vi "Elevator Controller.vi"(8 "error in":errorcluster) -> ()   [LabVIEW 2017]
doc: "This VI executes continuously carrying out the current operation and responding to updates or new operations. It will often contain the timing or control code that is difficult to place directly in TeleOp. This VI generally opens all sensors and motors and isolates the rest of the robot code from knowing how the operations are carried out."
uses:
  <vilib>/Rock Robotics/WPI/Framework/Completion Status.ctl
  Elevator Setpoints.ctl
  Elevator Operations.ctl
  <vilib>/Rock Robotics/WPI/ThirdParty/Phoenix-LabVIEW/Motor Controller/Controls/CTRE_Phoenix_MotorControl_FeedbackDevice.ctl
  <vilib>/Rock Robotics/WPI/ThirdParty/Phoenix-LabVIEW/Motor Controller/Controls/CTRE_Phoenix_MotorControl_LimitSwitchNormal.ctl
  <vilib>/Rock Robotics/WPI/ThirdParty/Phoenix-LabVIEW/Motor Controller/Controls/CTRE_Phoenix_MotorControl_LimitSwitchSource_Local.ctl
  <vilib>/Rock Robotics/WPI/ThirdParty/Phoenix-LabVIEW/Motor Controller/Controls/CTRE_Phoenix_MotorControl_ControlMode.ctl
  <vilib>/Rock Robotics/WPI/ThirdParty/Phoenix-LabVIEW/Motor Controller/Get/CTRE_Phoenix_MotorController_GetSelectedSensorData.vi
  <vilib>/Rock Robotics/Network Tables/NT Write Boolean.vi
panel:
  out "Position (Raw Sensor Units)":i32
  in  "Acceleration":i32
  in  "Cruise Velocity":i32
  in  "F":dbl
  in  "P":dbl
  in  "I":dbl
  in  "D":dbl
  in  "Interactive Values":T1
  out "Current\nCmd":string
  in  "Buttons":cluster{"Execute Cmd":bool, "Abort Cmd":bool}
  out "Command Timing":cluster{"Start Time (ms)":u32, "Iterations":i32}
  out "Status":T3
  # "Tip: It may be helpful to observe inputs and sensor values.\nYou may also want to display tuning or debugging controls."
  # "Interactive Command: You may fill in the settings for a command\nand schedule it with the Execute button. You can observe and abort\nany command while fine tuning the code for the controller."
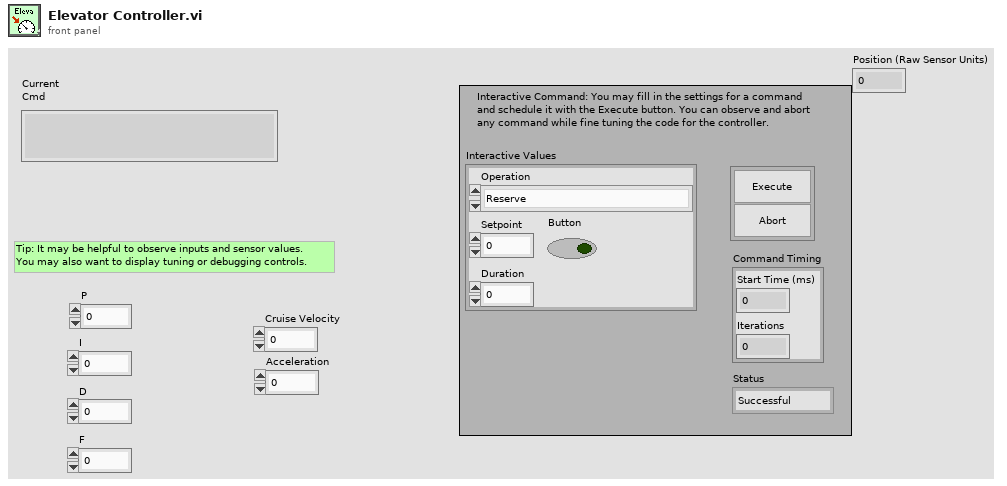
[diagram p1: front panel]
types:
  T1 = typedef "Elevator Setpoints.ctl" = cluster{"Operation":T2, "Setpoint":dbl, "Duration":dbl, "Button":bool}
  T2 = typedef "Elevator Operations.ctl" = enum16{"Reserve", "Read Current", "Immediate", "GoToHeight", "StayAtHeight", "LiftForTime"}
  T3 = typedef "Completion Status.ctl" = enum16{"Successful", "Aborted", "Incomplete"}
  T4 = typedef "CTRE_Phoenix_MotorControl_LimitSwitchSource_Local.ctl" = enum16{"Feedback Connector", "Remote Talon SRX", "Remote CANifier", "Deactivated"}
  T5 = typedef "CTRE_Phoenix_MotorControl_LimitSwitchNormal.ctl" = enum16{"Normally Open", "Normally Closed", "Disabled"}
  T6 = typedef "CTRE_Phoenix_MotorControl_FeedbackDevice.ctl" = i8
  T7 = typedef "WPI_MotorControlDeviceRef.ctl" = cluster{"DeviceStatus":errorcluster, "Type":T8, "PWM":cluster{"PWM Channel":T9, "DeadBand":T10}, "CAN":cluster{"Device Number":u8, "SetOutput VI Ref":variant, "GetOutput VI Ref":variant, "Enable VI Ref":variant, "Disable VI Ref":variant, "Data":variant}, "Invert":bool, "DIO PWM":cluster{"PWM \"Enable\" Channel":T9, "DIOChannel":T11, "PWM Rate":dbl}}
  T8 = typedef "WPI_MotorControlType.ctl" = enum16{"PWM", "CAN", "DIO PWM"}
  T9 = typedef "FPGA_DIOPWMChannel.ctl" = enum8{"PWM 0", "PWM 1", "PWM 2", "PWM 3", "PWM 4", "PWM 5", "PWM 6", "PWM 7", "PWM 8", "PWM 9", "PWM MXP 0", "PWM MXP 1", "PWM MXP 2", "PWM MXP 3", "PWM MXP 4", "PWM MXP 5", "PWM MXP 6", "PWM MXP 7", "PWM MXP 8", "PWM MXP 9", "Invalid"}
  T10 = typedef "WPI_PWMDeadband.ctl" = cluster{"Name":string, "maxPositivePwm":i32, "minPositivePwm":i32, "centerPwm":i32, "maxNegativePwm":i32, "minNegativePwm":i32, "angularRange":u16}
  T11 = typedef "FPGA_DIOChannel.ctl" = enum8{"DIO 0", "DIO 1", "DIO 2", "DIO 3", "DIO 4", "DIO 5", "DIO 6", "DIO 7", "DIO 8", "DIO 9", "DIO MXP 0", "DIO MXP 1", "DIO MXP 2", "DIO MXP 3", "DIO MXP 4", "DIO MXP 5", "DIO MXP 6", "DIO MXP 7", "DIO MXP 8", "DIO MXP 9", "DIO MXP 10", "DIO MXP 11", "DIO MXP 12", "DIO MXP 13", "DIO MXP 14", "DIO MXP 15", "SPI Port CS1", "SPI Port CS2", "SPI Port CS3", "SPI Port MISO", "SPI Port MOSI", "Invalid"}
  T12 = typedef "Command Status Info.ctl" = cluster{"Name":string, "Status":T3, "notifier out":T13}
  T13 = typedef "Completion Notifier.ctl" = refnum<notifier>
  T14 = cluster{"Current Command":T1, "Command Timing":cluster{"Start Time (ms)":u32, "Iterations":i32}, "Command Arguments":cluster{"Command Info":T12, "Description":string, "Default Command":T1, "queue out":refnum<queue>, "Subsystem Name":string}}
  T15 = typedef "CTRE_Phoenix_MotorControl_ControlMode.ctl" = u16
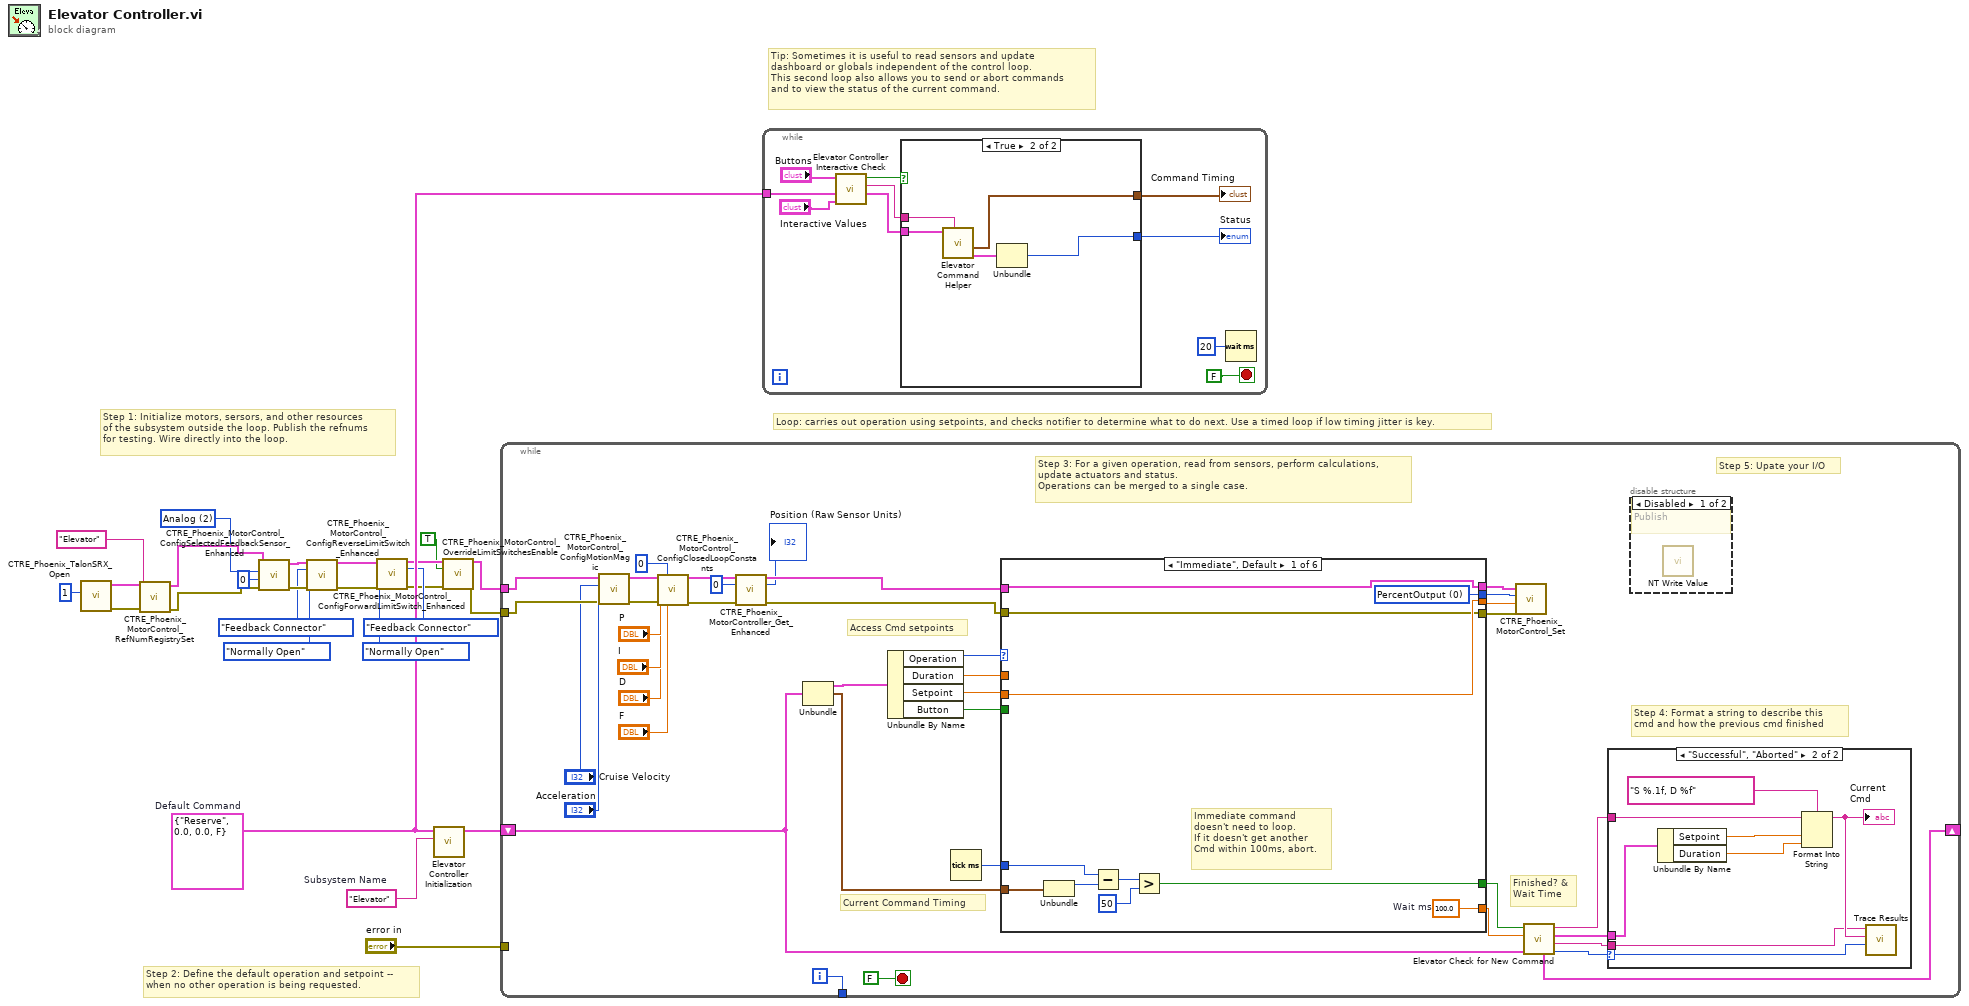
[diagram p0: block diagram]
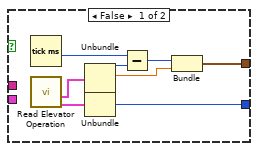
[diagram p2: hidden frame]
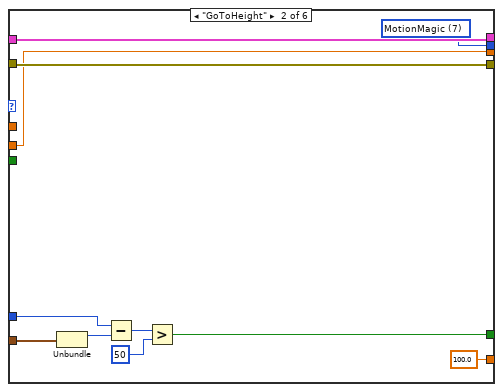
[diagram p5: hidden frame]
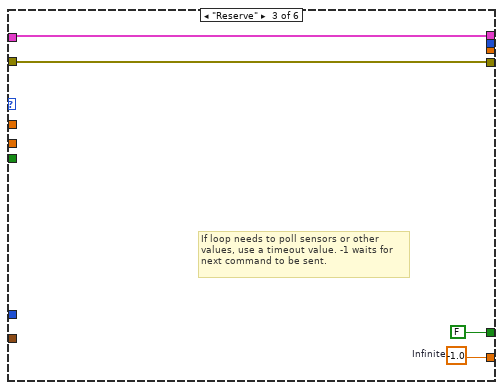
[diagram p6: hidden frame]
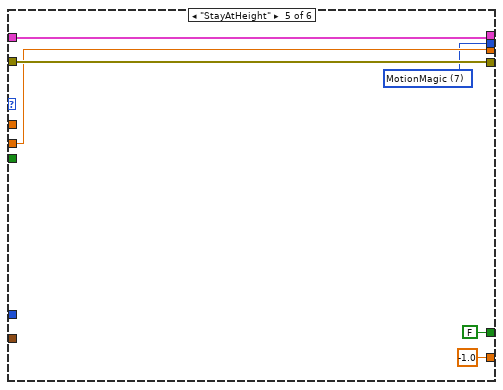
[diagram p8: hidden frame]
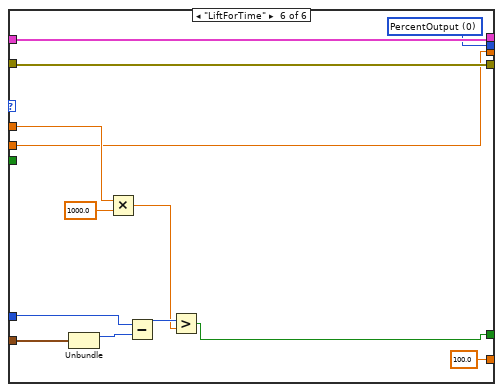
[diagram p9: hidden frame]
diagram:
  w15 = T6 2 items=["None"=-1, "QuadEncoder"=0, "Analog"=2, "Tachometer"=4, "Pulse Width Encoded Position"=8, "Sensor Sum (S0 + S1)"=9, "Sensor Difference (D0 - D1)"=10, "Remote Source 0"=11, "Remote Source 1"=12, "Software Emulated"=15] ("Feedback Device")
  w22 = T1 {"Operation"=enum."Reserve", "Setpoint"=0.0, "Duration"=0.0, "Button"=FALSE}  # Default Command
  w23 = "Elevator"  # Subsystem Name
  # "Tip: Sometimes it is useful to read sensors and update\ndashboard or globals independent of the control loop.\nThis second loop also allows you to send or abort commands\nand to view the status of the current command."
  # "Step 2: Define the default operation and setpoint --\nwhen no other operation is being requested."
  # "Step 1: Initialize motors, sersors, and other resources\nof the subsystem outside the loop. Publish the refnums\nfor testing. Wire directly into the loop."
  # "Loop: carries out operation using setpoints, and checks notifier to determine what to do next. Use a timed loop if low timing jitter is key."
  n1 = call <vilib>:"CTRE_Phoenix_TalonSRX_Open.vi"("Device Number"=u8 1) -> ("error out"=w20:errorcluster, "CAN Talon SRX Ref"=w21:T7)  [unwired: 9 in]
  n2 = call <vilib>:"CTRE_Phoenix_MotorControl_RefNumRegistrySet.vi"("error in (no error)"=w20, "refnum name"="Elevator", "PhoenixMotorControlDevRef"=w21) -> ("error out"=w17:errorcluster, "PhoenixMotorControlDevRef"=w16:T7)  [unwired: 7 in]
  n3 = call <vilib>:"CTRE_Phoenix_MotorControl_ConfigSelectedFeedbackSensor_Enhanced.vi"("error in (no error)"=w17, "pidLoopIdx"=0, "Feedback Device"=w15, "PhoenixMotorControlDevRef"=w16) -> ("error out"=w12:errorcluster, "PhoenixMotorControlDevRef"=w13:T7)  [unwired: 6 in]
  n4 = call <vilib>:"CTRE_Phoenix_MotorControl_ConfigReverseLimitSwitch_Enhanced.vi"("PhoenixMotorControlDevRef"=w13, "Limit Switch Source"=CTRE_Phoenix_MotorControl_LimitSwitchSource_Local."Feedback Connector", "NormallyOpenOrClosed"=CTRE_Phoenix_MotorControl_LimitSwitchNormal."Normally Open", "error in (no error)"=w12) -> ("PhoenixMotorControlDevRef"=w10:T7, "error out"=w11:errorcluster)  [unwired: 10 in]
  n5 = call <vilib>:"CTRE_Phoenix_MotorControl_ConfigForwardLimitSwitch_Enhanced.vi"("PhoenixMotorControlDevRef"=w10, "Limit Switch Source"=CTRE_Phoenix_MotorControl_LimitSwitchSource_Local."Feedback Connector", "NormallyOpenOrClosed"=CTRE_Phoenix_MotorControl_LimitSwitchNormal."Normally Open", "error in (no error)"=w11) -> ("PhoenixMotorControlDevRef"=w5:T7, "error out"=w4:errorcluster)  [unwired: 10 in]
  n6 = call "Elevator Controller Initialization.vi"("Subsystem Name"=w23, "Default Command"=w22) -> ("Current Command"=w24:T14)  [unwired: 9 in]
  n7 = call <vilib>:"CTRE_Phoenix_MotorControl_OverrideLimitSwitchesEnable.vi"("PhoenixMotorControlDevRef"=w5, "Override Limit Switch Enable?"=TRUE, "error in (no error)"=w4) -> ("PhoenixMotorControlDevRef"=w2:T7, "error out"=w1:errorcluster)  [unwired: 11 in]
  n8 = while {
    shift-right: [w56] -> _
    shift-left: w24 -> [w49]
    tunnel: [w62] -> _
    tunnel: "error in" -> [_]
    tunnel: w2 -> [w36]
    tunnel: w1 -> [w35]
    i -> [w62]
    stop <- FALSE stop-if-true
    # "Step 5: Upate your I/O"
    # "Step 4: Format a string to describe this\ncmd and how the previous cmd finished"
    # "Current Command Timing"
    # "Access Cmd setpoints"
    # "Finished? &\nWait Time"
    # "Step 3: For a given operation, read from sensors, perform calculations,\nupdate actuators and status.\nOperations can be merged to a single case."
    n9 = call <vilib>:"CTRE_Phoenix_MotorControl_ConfigMotionMagic.vi"("error in (no error)"=w35, "Acceleration"="Acceleration", "Cruise Velocity"="Cruise Velocity", "PhoenixMotorControlDevRef"=w36) -> ("error out"=w41:errorcluster, "PhoenixMotorControlDevRef"=w40:T7)  [unwired: 6 in]
    n10 = call <vilib>:"CTRE_Phoenix_MotorControl_ConfigClosedLoopConstants.vi"("PhoenixMotorControlDevRef"=w40, "slotIdx"=0, "P"="P", "I"="I", "D"="D", "error in (no error)"=w41, "F"="F") -> ("PhoenixMotorControlDevRef"=w31:T7, "error out"=w30:errorcluster)  [unwired: 7 in]
    n11 = call-poly <vilib>:"CTRE_Phoenix_MotorController_Get_Enhanced.vi"("PhoenixMotorControlDevRef"=w31, "pidLoopIdx"=u32 0, "error in"=w30) -> ("PhoenixMotorControlDevRef"=w29:T7, "Position (Raw Sensor Units)"=→"Position (Raw Sensor Units)":i32, "error out"=w28:errorcluster)  [unwired: 9 in, 1 out]
    n12 = Unbundle(w49) -> ("Current Command"=w61:T1, "Command Timing"=w58:cluster{"Start Time (ms)":u32, "Iterations":i32})  [unwired: 1 out]
    n13 = Unbundle By Name(w61) -> ("Operation"=w60:T2, "Duration"=w59:dbl, "Setpoint"=w57:dbl, "Button"=w33:bool)
    n14 = Tick Count (ms)() -> (millisecond timer value=w48:u32)
    n15 = case shown="\"Immediate\", Default" w60 {
      tunnel: [w82 100.0 ("Infinite") w97 _ -1.0 ("Infinite") 100.0 ("Infinite")] -> w54
      tunnel: [w76 w88 FALSE ("ignore previous (F)") _ FALSE ("ignore previous (F)") w111] -> w55
      tunnel: w58 -> [w78 w89 _ _ _ w112]
      tunnel: w59 -> [_ _ _ _ _ w109]
      tunnel: w57 -> [w74 w85 _ _ w103 w106]
      tunnel: w29 -> [w72 w87 w95 w99 w105 w118]
      tunnel: w28 -> [w73 w86 w94 w98 w104 w117]
      tunnel: w48 -> [w77 w90 _ _ _ w113]
      tunnel: [w73 w86 w94 w98 w104 w117] -> w47
      tunnel: [w72 w87 w95 w99 w105 w118] -> w46
      tunnel: [w74 w85 _ _ w103 w106] -> w45
      tunnel: [w75 w84 _ _ w101 w116] -> w34
      tunnel: w33 -> [_ _ _ _ _ _]
      frame "Immediate", Default {
        w75 = T15 0 items=["PercentOutput"=0, "Position"=1, "Velocity"=2, "Current"=3, "Follower"=5, "MotionProfile"=6, "MotionMagic"=7, "MotionMagicArc"=8, "MotionProfileArc"=10, "Disabled"=15] ("Control Mode")
        w82 = 100.0  # Wait ms
        # "Immediate command\ndoesn't need to loop.\nIf it doesn't get another\nCmd within 100ms, abort."
        n16 = Unbundle(w78) -> ("Start Time (ms)"=w81:u32)  [unwired: 1 out]
        n17 = Subtract(x=w77, y=w81) -> (x-y=w80:u32)
        n18 = Greater?(x=w80, y=u8 50 ("Left Motor")) -> (0:w76:bool)
      }
      frame "GoToHeight" {
        w84 = T15 7 items=["PercentOutput"=0, "Position"=1, "Velocity"=2, "Current"=3, "Follower"=5, "MotionProfile"=6, "MotionMagic"=7, "MotionMagicArc"=8, "MotionProfileArc"=10, "Disabled"=15] ("Control Mode")
        n19 = Unbundle(w89) -> ("Start Time (ms)"=w93:u32)  [unwired: 1 out]
        n20 = Subtract(x=w90, y=w93) -> (x-y=w92:u32)
        n21 = Greater?(x=w92, y=u8 50 ("Left Motor")) -> (0:w88:bool)
      }
      frame "Reserve" {
        w97 = -1.0  # Infinite
        # "If loop needs to poll sensors or other\nvalues, use a timeout value. -1 waits for\nnext command to be sent."
      }
      frame "Read Current" {
      }
      frame "StayAtHeight" {
        w101 = T15 7 items=["PercentOutput"=0, "Position"=1, "Velocity"=2, "Current"=3, "Follower"=5, "MotionProfile"=6, "MotionMagic"=7, "MotionMagicArc"=8, "MotionProfileArc"=10, "Disabled"=15] ("Control Mode")
      }
      frame "LiftForTime" {
        w116 = T15 0 items=["PercentOutput"=0, "Position"=1, "Velocity"=2, "Current"=3, "Follower"=5, "MotionProfile"=6, "MotionMagic"=7, "MotionMagicArc"=8, "MotionProfileArc"=10, "Disabled"=15] ("Control Mode")
        n22 = Unbundle(w112) -> ("Start Time (ms)"=w114:u32)  [unwired: 1 out]
        n23 = Multiply(x=w109, y=1000.0) -> (x*y=w108:dbl)
        n24 = Subtract(x=w113, y=w114) -> (x-y=w115:u32)
        n25 = Greater?(x=w115, y=w108) -> (0:w111:bool)
      }
    }
    n26 = call <vilib>:"CTRE_Phoenix_MotorControl_Set.vi"("error in (no error)"=w47, "Output"=w45, "Control Mode"=w34, "PhoenixMotorControlDevRef"=w46) -> ()  [unwired: 6 in, 2 out]
    n27 = call "Elevator Check for New Command.vi"("Current Command"=w49, "Wait time (ms)"=w54, "Finished?"=w55) -> ("Completion"=w50:T3, "Subsystem Name"=w51:string, "Current Command"=w52:T1, "Initial Trace String"=w53:string, "NextCommand"=w56:T14)  [unwired: 4 in]
    n28 = case shown="\"Successful\", \"Aborted\"" w50 {
      selector: w50 -> [_ w71]
      tunnel: w53 -> [_ w67]
      tunnel: w52 -> [_ w68]
      tunnel: w51 -> [_ w64]
      frame "Incomplete", Default {
        # "Continuing current command"
      }
      frame "Successful", "Aborted" {
        # "Report and setup for next command"
        n29 = Unbundle By Name(w68) -> ("Setpoint"=w70:dbl, "Duration"=w65:dbl)
        n30 = Format Into String(format string="S %.1f, D %f", initial string=w67, w70, w65) -> (resulting string=w66:string)  [unwired: 1 in, 1 out]
        "Current\nCmd" <- w66
        n31 = call <vilib>:"Trace Results.vi"("Status of previous command"=w71, "Description"=w66, "Subsystem"=w64) -> ()  [unwired: 9 in]
      }
    }
    n32 = disable-structure shown="Disabled" {
      frame Disabled {
        # "Publish"
        n33 = call-poly <vilib>:"NT Write Value.vi"() -> ()  [unwired: 11 in, 1 out]
      }
      frame Enabled {
      }
    }
  }
  n34 = while {
    tunnel: w22 -> [w125]
    stop <- FALSE stop-if-true
    n35 = call "Elevator Controller Interactive Check.vi"("Interactive Command in"="Interactive Values", "Default Command"=w125, "Buttons"="Buttons") -> ("Interactive Command out"=w122:T1, "Trace String"=w123:string, "Schedule"=w124:bool)  [unwired: 6 in]
    n36 = case shown="True" w124 {
      tunnel: [w136 w141] -> w121
      tunnel: w122 -> [_ w139]
      tunnel: [w132 w137] -> w120
      tunnel: w123 -> [_ w140]
      frame False {
        n37 = Tick Count (ms)() -> (millisecond timer value=w131:u32)
        n38 = call "Read Elevator Operation.vi"() -> ("Command Info"=w129:T12, "SubSystem Data"=w130:T1)  [unwired: 9 in, 1 out]
        n39 = Unbundle(w130) -> ("Operation"=w135:T2, "Setpoint"=w133:dbl)  [unwired: 2 out]
        n40 = Unbundle(w129) -> ("Status"=w136:T3)  [unwired: 2 out]
        n41 = Subtract(x=w131, y=w135) -> (x-y=w134:u32)
        n42 = Bundle(w134, "Setpoint"=w133) -> (w132:cluster{u32, "Setpoint":dbl})  [unwired: 1 in]
      }
      frame True {
        n43 = call "Elevator Command Helper.vi"("Description"=w140, "SubSystem Data"=w139) -> ("Command Info Out"=w138:T12, "Command Timing"=w137:cluster{"Start Time (ms)":u32, "Iterations":i32})  [unwired: 7 in, 1 out]
        n44 = Unbundle(w138) -> ("Status"=w141:T3)  [unwired: 2 out]
      }
    }
    "Status" <- w121
    "Command Timing" <- w120
    n45 = Wait (ms)(milliseconds to wait=u32 20) -> ()  [unwired: 1 out]
  }
